vi "Stop (FGV).vi"(7 "Enum(read)":enum16{"write", "read"}(ring)=enum."read", 8 "error in (no error)":errorcluster, 10 "Stop in":bool) -> (0 "error out":errorcluster, 2 "Stop out":bool)   [LabVIEW 2018]
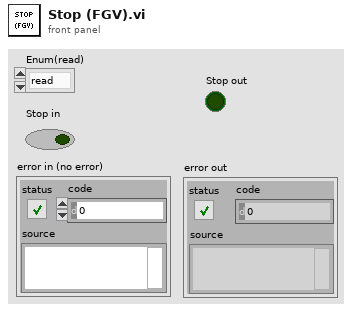
[diagram p1: front panel]
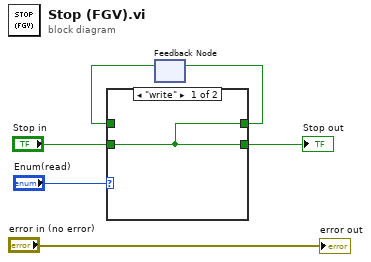
[diagram p0: block diagram]
diagram:
  n1 = feedback #1() -> (w1:bool)  [unwired: 1 in]
  n2 = case shown="\"write\"" "Enum(read)" {
    tunnel: "Stop in" -> [w7 _]
    tunnel: [w7 w8] -> w2
    tunnel: w1 -> [_ w8]
    tunnel: [w7 w8] -> w4
    frame "write" {
    }
    frame "read", Default {
    }
  }
  "Stop out" <- w4
  n3 = feedback-in #1(w2) -> ()
  "error out" <- "error in (no error)"
